vi "Calc Plot.vi"(0 "DataSets":T1 {"Deltas(PPM)" format="%.8f"; "Frequency(Hz)" format="%.2f"; "Time" format="%.2f"}, 1 "error in (no error)":errorcluster) -> (2 "Elapsed Time":dbl format="%.2f", 3 "Plot Data":cluster{dbl[], dbl[]} {"?" format="%.2f"; "?" format="%.2f"}, 4 "Max Delta":dbl format="%.2f")   [LabVIEW 2021]
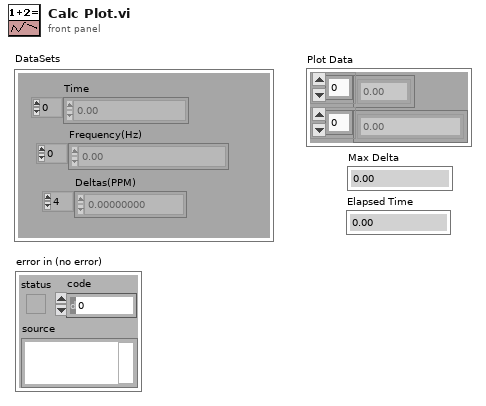
[diagram p1: front panel]
types:
  T1 = cluster{"Time":dbl[], "Frequency(Hz)":dbl[], "Deltas(PPM)":dbl[]}
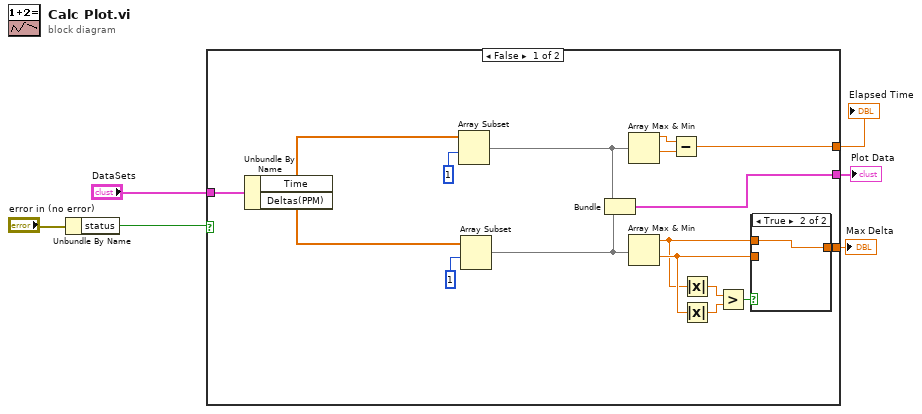
[diagram p0: block diagram]
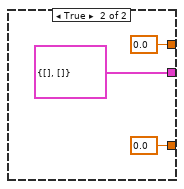
[diagram p3: hidden frame]
diagram:
  n1 = Unbundle By Name("error in (no error)") -> ("status"=w1:bool)
  n2 = case shown="False" w1 {
    tunnel: [w21 0.0] -> w6
    tunnel: [w18 0.0] -> w5
    tunnel: [w10 cluster{dbl[], dbl[]} {[], []}] -> w4
    tunnel: "DataSets" -> [w9 _]
    frame False {
      n3 = Unbundle By Name(w9) -> ("Time"=w8:dbl[], "Deltas(PPM)"=w7:dbl[])
      n4 = Array Subset(array=w8, index=1) -> (w14:dbl[])  [unwired: 1 in]
      n5 = Array Subset(array=w7, index=1) -> (w12:dbl[])  [unwired: 1 in]
      n6 = Bundle(w14, w12) -> (w10:cluster{dbl[], dbl[]})  [unwired: 1 in]
      n7 = Array Max & Min(array=w14) -> (max value=w22:dbl, min value=w23:dbl)  [unwired: 2 out]
      n8 = Array Max & Min(array=w12) -> (max value=w19:dbl, min value=w20:dbl)  [unwired: 2 out]
      n9 = Subtract(x=w22, y=w23) -> (x-y=w21:dbl)
      n10 = Absolute Value(x=w19) -> (abs(x)=w16:dbl)
      n11 = Absolute Value(x=w20) -> (abs(x)=w15:dbl)
      n12 = Greater?(x=w16, y=w15) -> (0:w17:bool)
      n13 = case shown="True" w17 {
        tunnel: w19 -> [_ w25]
        tunnel: w20 -> [w24 _]
        tunnel: [w24 w25] -> w18
        frame False {
        }
        frame True {
        }
      }
    }
    frame True {
    }
  }
  "Elapsed Time" <- w6
  "Max Delta" <- w5
  "Plot Data" <- w4
